vi "数组值的范围子VI.vi"(3 "下限":dbl, 4 "数组":dbl[][](array[numeric]), 5 "上限":dbl) -> (1 "数组 2":dbl[][](array[numeric]))   [LabVIEW 2013]
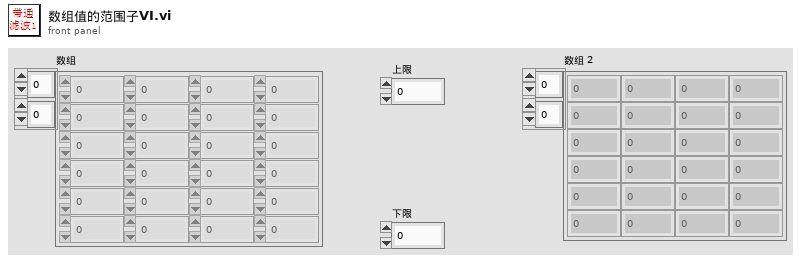
[diagram p1: front panel]
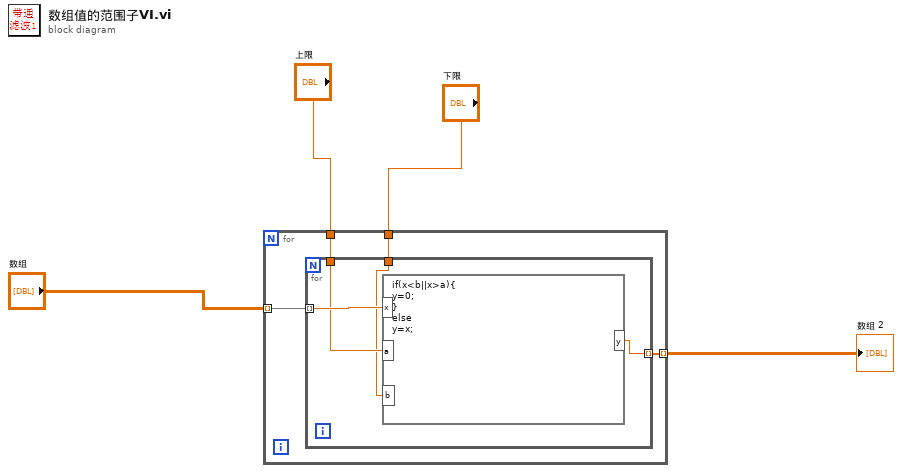
[diagram p0: block diagram]
diagram:
  n1 = for {
    tunnel: "数组" -> [w8] mode=indexing
    tunnel: [w7] -> w3 mode=indexing
    tunnel: "上限" -> [w6]
    tunnel: "下限" -> [w5]
    n2 = for {
      tunnel: w8 -> [w12] mode=indexing
      tunnel: [w11] -> w7 mode=indexing
      tunnel: w6 -> [w10]
      tunnel: w5 -> [w9]
      n3 = formula code="if(x<b||x>a){\ny=0;\n}\nelse\ny=x;"("x"=w12, "a"=w10, "b"=w9) -> ("y"=w11:dbl)
    }
  }
  "数组 2" <- w3
